vi "Z900_navX_Util_EncodeProtocol_SignedRatio.vi"(1 "Signed Ratio":dbl[](array[numeric])) -> (0 "Little Endian":u8[](array[numeric]))   [LabVIEW 2015, in "Apple Pi Gyro Library.lvlib" / "navX Library v2.lvlib"]
uses:
  navX Library v2.lvlib
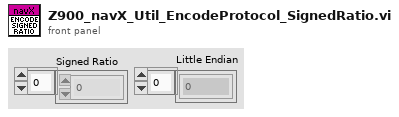
[diagram p1: front panel]
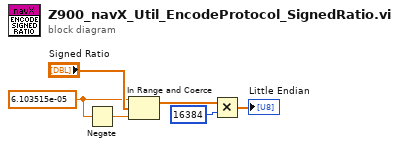
[diagram p0: block diagram]
diagram:
  w3 = 6.103515e-05
  n1 = Negate(x=w3) -> (-x=w2:dbl)
  n2 = In Range and Coerce(upper limit=w3, x="Signed Ratio", lower limit=w2) -> (coerced(x)=w1:dbl[])  [unwired: 1 out]
  n3 = Multiply(x=w1, y=u16 16384) -> (x*y=→"Little Endian":dbl[])
